vi "时间字符串至时间格式转换.vi"(11 "字符串":string) -> (3 "seconds since 1Jan1904":timestamp)   [LabVIEW 2016, in "超标留样集成.lvlib" / "科盛超标留样.lvlib"]
uses:
  <vilib>/Utility/miscctls.llb/LVDateTimeRec.ctl
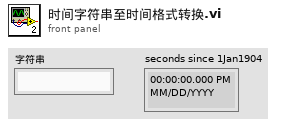
[diagram p1: front panel]
types:
  T1 = typedef "LVDateTimeRec.ctl" = cluster{"fractional second":dbl, "second":i32, "minute":i32, "hour":i32, "day of month":i32, "month":i32, "year":i32, "day of week":i32, "day of year":i32, "DST":i32}
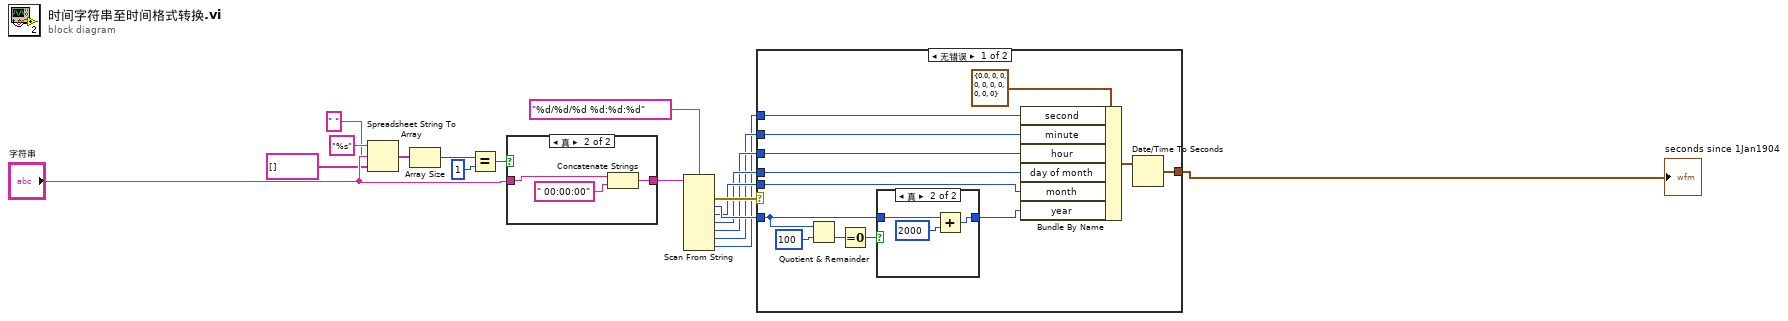
[diagram p0: block diagram]
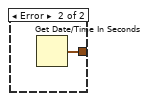
[diagram p4: hidden frame]
diagram:
  n1 = Spreadsheet String To Array(delimiter (Tab)=" " ("分隔符(Tab)"), format string="%s" ("格式字符串"), spreadsheet string="字符串", array type (2D Dbl)=string[] []) -> (array=w12:string[])
  n2 = Array Size(array=w12) -> (size(s)=w13:i32)
  n3 = Equal?(x=w13, y=1) -> (x = y?=w15:bool)
  n4 = case shown="真" w15 {
    tunnel: "字符串" -> [w19 w21]
    tunnel: [w19 w20] -> w16
    frame False {
    }
    frame True {
      n5 = Concatenate Strings(w21, " 00:00:00" ("字符串")) -> (w20:string)
    }
  }
  n6 = Scan From String(format string="%d/%d/%d %d:%d:%d" ("格式字符串"), input string=w16) -> (error out=w8:errorcluster, output 1=w6:i32, output 2=w5:i32, output 3=w4:i32, output 4=w3:i32, output 5=w2:i32, output 6=w1:i32)  [unwired: 8 in, 2 out]
  n7 = case shown="无错误" w8 {
    tunnel: w1 -> [w34 _]
    tunnel: w2 -> [w33 _]
    tunnel: w3 -> [w32 _]
    tunnel: w4 -> [w31 _]
    tunnel: w5 -> [w30 _]
    tunnel: w6 -> [w26 _]
    tunnel: [w28 w40] -> w18
    frame No Error {
      n8 = Quotient & Remainder(x=w26, y=100) -> (floor(x/y)=w25:i32)  [unwired: 1 out]
      n9 = Equal To 0?(x=w25) -> (x = 0?=w24:bool)
      n10 = case shown="真" w24 {
        tunnel: w26 -> [w36 w39]
        tunnel: [w36 w37] -> w23
        frame False {
        }
        frame True {
          n11 = Add(x=w39, y=2000) -> (x+y=w37:i32)
        }
      }
      n12 = Bundle By Name(cluster=T1 {"fractional second"=0.0, "second"=0, "minute"=0, "hour"=0, "day of month"=0, "month"=0, "year"=0, "day of week"=0, "day of year"=0, "DST"=0} ("日期时间记录"), "second"=w34, "minute"=w33, "hour"=w32, "day of month"=w31, "month"=w30, "year"=w23) -> (w35:T1)
      n13 = Date/Time To Seconds(2:w35) -> (0:w28:timestamp)  [unwired: 1 in]
    }
    frame Error {
      n14 = Get Date/Time In Seconds() -> (seconds since 1Jan1904=w40:timestamp)
    }
  }
  "seconds since 1Jan1904" <- w18
